vi "USRP (transmitter,9600,repeatition).vi"() -> ()   [LabVIEW 2013]
uses:
  IS-95/transmitter/4800/coding(4800).vi
  IS-95/transmitter/common/interleaver.vi
  IS-95/transmitter/9600/coding(9600).vi
  <vilib>/Analysis/baseanly.llb/A x B.vi
  <vilib>/Analysis/baseanly.llb/Real A x B.vi
  IS-95/transmitter/4800/syndrom(4800).vi
  IS-95/transmitter/9600/syndrom(9600).vi
  <vilib>/Analysis/Matrix/Numeric/Conversions/Array To Matrix.vi
  <vilib>/Analysis/Matrix/Numeric/Conversions/Array To Matrix - RA.vi
  <instrlib>/niUSRP/niUSRP Write Tx Data (CDB).vi
panel:
  in  "num of channels":i32=63
  in  "IQ rate":dbl=850000.0 format="%#_13g"
  out "transmitted bits":bool[][](array[boolean])
  in  "device name":refnum<k15>="192.168.10.3"
  in  "gain":dbl format="%#_6f"
  in  "carrier freq.":dbl=850000000.0 format="%#_6p"
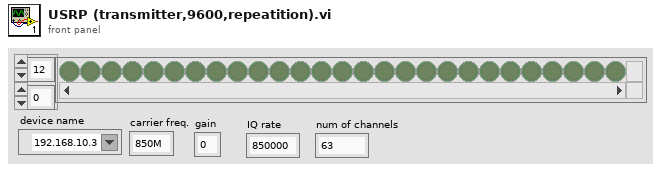
[diagram p1: front panel]
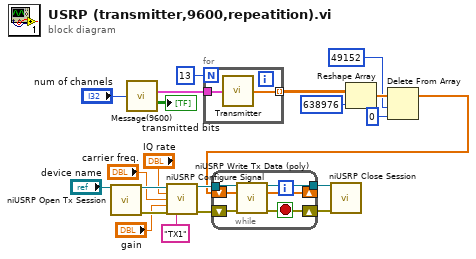
[diagram p0: block diagram]
diagram:
  n1 = call <instrlib>:"niUSRP Open Tx Session.vi"("device names"="device name") -> ("session handle out"=w21:refnum<k15>, "error out"=w20:errorcluster)  [unwired: 13 in]
  n2 = call "Message(9600).vi"("Число каналов"="num of channels") -> ("Channels"=w8:cluster{dbl, i32, bool[], "Type":i32}[], "Message"=→"transmitted bits":bool[][])  [unwired: 13 in]
  n3 = call <instrlib>:"niUSRP Configure Signal.vi"("session handle"=w21, "IQ rate"="IQ rate", "carrier frequency"="carrier freq.", "gain"="gain", "error in (no error)"=w20, "active antenna"="TX1") -> ("session handle out"=w14:refnum<k15>, "error out"=w13:errorcluster)  [unwired: 5 in, 3 out]
  n4 = for {
    N: 13 -> [_]
    tunnel: w8 -> [w23]
    tunnel: [w22] -> w7 mode=indexing
    n5 = call "Transmitter.vi"("CHANNELS"=w23) -> ("x + iy"=w22:cdb[])  [unwired: 14 in]
  }
  n6 = Reshape Array(w7, 638976 ("dimension size")) -> (w5:cdb[])
  n7 = Delete From Array(array=w5, length=49152, index=0) -> (array with subset deleted=w2:cdb[])  [unwired: 1 out]
  n8 = while {
    tunnel: w14 -> [w28]
    shift-right: [w25] -> w11
    shift-left: w13 -> [w26]
    tunnel: [w27] -> w12
    shift-right: [w24] -> _
    shift-left: w2 -> [w24]
    stop <- w25 stop-if-true
    n9 = call-poly <instrlib>:"niUSRP Write Tx Data (poly).vi"("session handle"=w28, "data"=w24, "error in (no error)"=w26) -> ("session handle out"=w27:refnum<k15>, "error out"=w25:errorcluster)  [unwired: 11 in]
  }
  n10 = call <instrlib>:"niUSRP Close Session.vi"("session handle"=w12, "error in (no error)"=w11) -> ()  [unwired: 13 in, 1 out]
